vi "TEST_Garaje.vi"() -> ()   [LabVIEW 2019]
uses:
  <vilib>/MakerHub/LINX/Public/Peripherals/Digital/Digital Read N Chans.vi
  <vilib>/MakerHub/LINX/Public/Peripherals/Digital/Digital Write N Chans.vi
  <vilib>/MakerHub/LINX/Public/Peripherals/Analog/Analog Read 1 Chan.vi
  <vilib>/MakerHub/LINX/Private/Local IO/LinxDigitalRead.vi
  <vilib>/MakerHub/LINX/Public/Utilities/Check Channel.vi
  <vilib>/MakerHub/LINX/Private/Local IO/LinxDigitalWrite.vi
  <vilib>/MakerHub/LINX/Public/Peripherals/Analog/Analog Read N Chans.vi
  <vilib>/MakerHub/LINX/Private/Local IO/LinxAnalogRead.vi
  <vilib>/MakerHub/LINX/Public/Utilities/Open Serial.vi
  <vilib>/MakerHub/LINX/Public/Sensors/Motion/Servo/Servo Open One Channel.vi
  <vilib>/MakerHub/LINX/Private/Utilties/Generate Error.vi
  <vilib>/MakerHub/LINX/Public/Sensors/Motion/Servo/Servo Set Pulse Width One Channel.vi
  <vilib>/MakerHub/LINX/Public/Sensors/Motion/Servo/Servo Close One Channel.vi
  <vilib>/MakerHub/LINX/LMH-LINX.lvlib
  <vilib>/MakerHub/LINX/Public/Sensors/Motion/Servo/Servo.lvlib
panel:
  out "Slide 2":dbl(slide) scale=0.0..5.0
  out "Voltaje LDR":dbl
  out "ROJO":bool
  out "VERDE":bool
  in  "Serial Port":refnum<visa-resource-name>
  out "Loop Rate (Hz)":u32
  in  "Abrir":bool
  in  "Cerrar":bool
  in  "Stop Button":bool
  out "Slide":i32(slide) scale=0.0..100.0
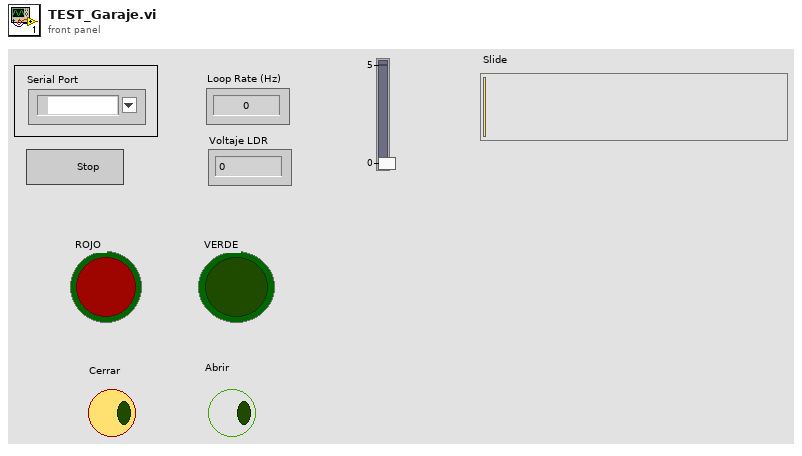
[diagram p1: front panel]
types:
  T1 = typedef "LMH-LINX.lvlib/LINX Ref.ctl" = cluster{"IO":T2, "Interface":T3, "LINX Device Config":T4}
  T2 = typedef "LMH-LINX.lvlib/Platform.ctl" = enum16{"Remote", "Local"}
  T3 = typedef "LMH-LINX.lvlib/Interface.ctl" = enum16{"Serial", "TCP"}
  T4 = typedef "LMH-LINX.lvlib/Device.lvlib/LINX Device Config.ctl" = cluster{"Interface":T3, "COM Port":refnum<visa-resource-name>, "TCP Configuration":T5, "Device Family":u8, "Device ID":u8, "Device Name":string, "TCP Ref":refnum<k5>, "Channels":T6}
  T5 = typedef "LMH-LINX.lvlib/Device.lvlib/TCP Config.ctl" = cluster{"IP Address":string, "Port":u16}
  T6 = typedef "LMH-LINX.lvlib/Channels.ctl" = cluster{"DI":u8[], "DO":u8[], "AI":u8[], "AO":u8[], "PWM":u8[], "QE":u8[], "UART":u8[], "I2C 2":u8[], "SPI":u8[], "CAN":u8[], "Servo":u8[], "AI Ref (V)":dbl, "AI Resolution (Bits)":u8, "AO Ref (V)":dbl, "AO Resolution (Bits)":u8}
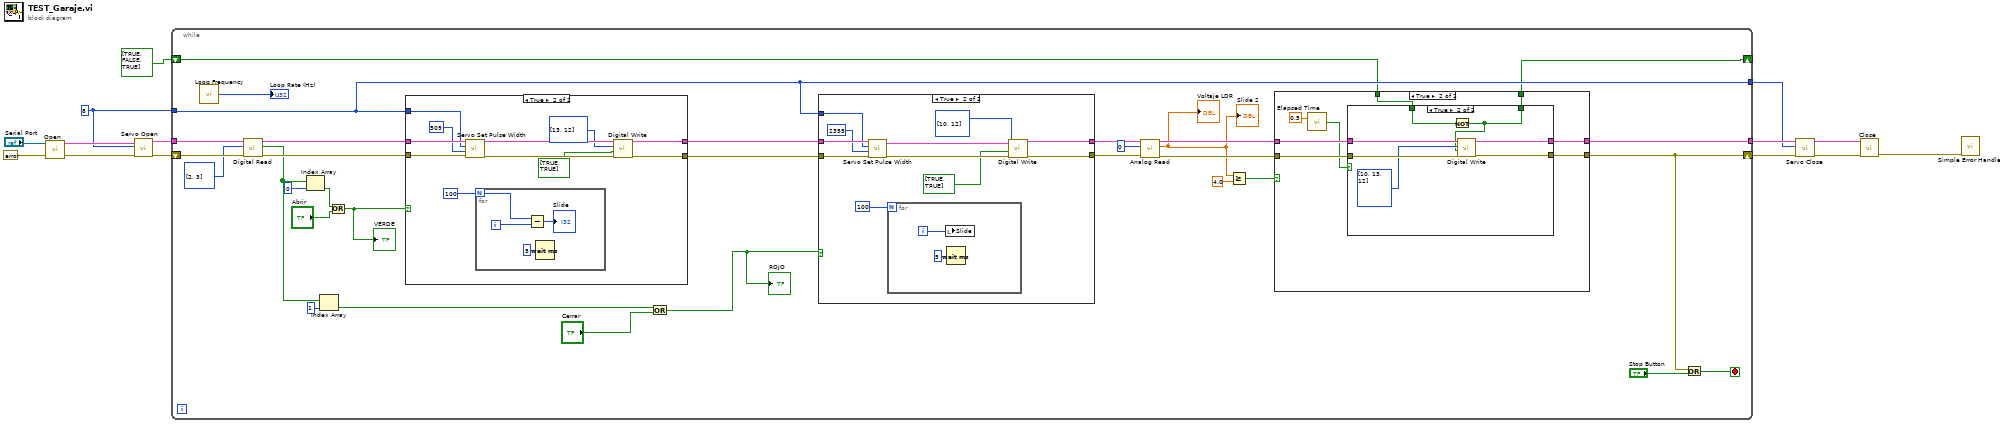
[diagram p0: block diagram]
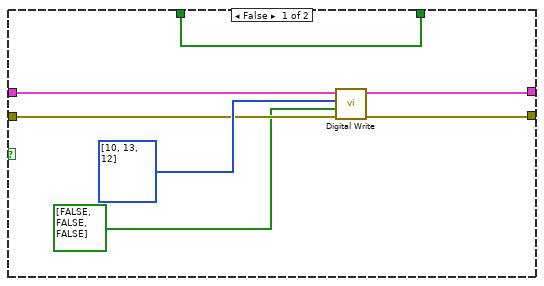
[diagram p2: hidden frame]
diagram:
  w4 = u8 8 ("Servo Channel")
  n1 = call-poly <vilib>:"Open.vi"("Error In"=errorcluster {"status"=FALSE, "code"=0, "source"=""}, "Serial Port"="Serial Port") -> ("Error Out"=w3:errorcluster, "LINX Resource"=w6:T1)  [unwired: 7 in, 1 out]
  n2 = call-poly <vilib>:"Servo Open.vi"("Error In"=w3, "Servo Channel"=w4, "LINX Resource"=w6) -> ("Error Out"=w2:errorcluster, "LINX Resource"=w5:T1)  [unwired: 7 in]
  n3 = while {
    tunnel: w5 -> [w39]
    shift-right: [w19] -> w10
    shift-left: w2 -> [w40]
    tunnel: w4 -> [w41]
    tunnel: [w20] -> w11
    tunnel: [w41] -> w7
    shift-right: [w16] -> _
    shift-left: bool[] [TRUE, FALSE, TRUE] ("Values") -> [w17]
    stop <- w46 stop-if-true
    n4 = call <vilib>:"Loop Frequency.vi"() -> ("Loop Rate (Hz)"=→"Loop Rate (Hz)":u32)
    n5 = call-poly <vilib>:"Digital Read.vi"("Error In"=w40, "DI Channels"=u8[] [2, 3] ("Array"), "LINX Resource"=w39) -> ("Error Out"=w37:errorcluster, "Values"=w32:bool[], "LINX Resource"=w38:T1)  [unwired: 6 in]
    n6 = Index Array "Index Array"(array=w32, index=0) -> (element=w33:bool)
    n7 = Index Array "Index Array"(array=w32, index=1) -> (element=w30:bool)
    n8 = Or(x=w33, y="Abrir") -> (x .or. y?=w28:bool)
    "VERDE" <- w28
    n9 = case shown="True" w28 {
      tunnel: w37 -> [w87 w99]
      tunnel: [w87 w92] -> w43
      tunnel: w38 -> [w88 w98]
      tunnel: [w88 w93] -> w42
      tunnel: w41 -> [_ w97]
      frame False {
      }
      frame True {
        n10 = call-poly <vilib>:"Servo Set Pulse Width.vi"("Error In"=w99, "Pulse Width (uS)"=509, "Servo Channel"=w97, "LINX Resource"=w98) -> ("Error Out"=w94:errorcluster, "LINX Resource"=w95:T1)  [unwired: 6 in]
        n11 = for {
          N: 100 -> [w103]
          i -> [w102]
          n12 = Subtract(x=w103, y=w102) -> (x-y=→"Slide":i32)
          n13 = Wait (ms)(milliseconds to wait=u32 5) -> ()  [unwired: 1 out]
        }
        n14 = call-poly <vilib>:"Digital Write.vi"("Error In"=w94, "Values"=bool[] [TRUE, TRUE], "DO Channels"=u8[] [13, 12], "LINX Resource"=w95) -> ("Error Out"=w92:errorcluster, "LINX Resource"=w93:T1)  [unwired: 6 in]
      }
    }
    n15 = Or(x=w30, y="Cerrar") -> (x .or. y?=w27:bool)
    "ROJO" <- w27
    n16 = case shown="True" w27 {
      tunnel: w43 -> [w72 w84]
      tunnel: [w72 w78] -> w25
      tunnel: w42 -> [w73 w83]
      tunnel: [w73 w77] -> w26
      tunnel: w41 -> [_ w82]
      frame False {
      }
      frame True {
        n17 = call-poly <vilib>:"Servo Set Pulse Width.vi"("Error In"=w84, "Pulse Width (uS)"=2355, "Servo Channel"=w82, "LINX Resource"=w83) -> ("Error Out"=w79:errorcluster, "LINX Resource"=w80:T1)  [unwired: 6 in]
        n18 = for {
          N: u8 100 ("Slide") -> [_]
          i -> [w85]
          n19 = local write "Slide"(w85) -> ()
          n20 = Wait (ms)(milliseconds to wait=u32 5) -> ()  [unwired: 1 out]
        }
        n21 = call-poly <vilib>:"Digital Write.vi"("Error In"=w79, "Values"=bool[] [TRUE, TRUE], "DO Channels"=u8[] [10, 12], "LINX Resource"=w80) -> ("Error Out"=w78:errorcluster, "LINX Resource"=w77:T1)  [unwired: 6 in]
      }
    }
    n22 = call-poly <vilib>:"Analog Read.vi"("Error In"=w25, "Analog Channel"=u8 0, "LINX Resource"=w26) -> ("Error Out"=w21:errorcluster, "Voltage"=w18:dbl, "LINX Resource"=w22:T1)  [unwired: 5 in, 1 out]
    "Voltaje LDR" <- w18
    "Slide 2" <- w18
    n23 = Greater Or Equal?(x=w18, y=4.0) -> (x >= y?=w15:bool)
    n24 = case shown="True" w15 {
      tunnel: w22 -> [w50 w60]
      tunnel: w21 -> [w51 w61]
      tunnel: [w49 w59] -> w20
      tunnel: [w48 w58] -> w19
      tunnel: w17 -> [w53 w57]
      tunnel: [w53 w56] -> w16
      frame False {
        n25 = call-poly <vilib>:"Digital Write.vi"("Error In"=w51, "Values"=bool[] [FALSE, FALSE, FALSE], "DO Channels"=u8[] [10, 13, 12] ("Array"), "LINX Resource"=w50) -> ("Error Out"=w48:errorcluster, "LINX Resource"=w49:T1)  [unwired: 6 in]
      }
      frame True {
        n26 = call "Elapsed Time"("Time Target (s)"=0.5) -> ("Time has Elapsed"=w54:bool)  [unwired: 11 in, 7 out]
        n27 = case shown="True" w54 {
          tunnel: w61 -> [w62 w71]
          tunnel: w60 -> [w63 w70]
          tunnel: [w63 w69] -> w59
          tunnel: [w62 w68] -> w58
          tunnel: w57 -> [w64 w66]
          tunnel: [w64 w65] -> w56
          frame False {
          }
          frame True {
            n28 = Not(x=w66) -> (.not. x?=w65:bool[])
            n29 = call-poly <vilib>:"Digital Write.vi"("Error In"=w71, "Values"=w65, "DO Channels"=u8[] [10, 13, 12] ("Array"), "LINX Resource"=w70) -> ("Error Out"=w68:errorcluster, "LINX Resource"=w69:T1)  [unwired: 6 in]
          }
        }
      }
    }
    n30 = Or(x=w19, y="Stop Button") -> (x .or. y?=w46:bool)
  }
  n31 = call-poly <vilib>:"Servo Close.vi"("Error In"=w10, "Servo Channel"=w7, "LINX Resource"=w11) -> ("Error Out"=w9:errorcluster, "LINX Resource"=w8:T1)  [unwired: 7 in]
  n32 = call <vilib>:"Close.vi"("Error In"=w9, "LINX Resource"=w8) -> ("Error Out"=w14:errorcluster)  [unwired: 9 in]
  n33 = call <vilib>:"Simple Error Handler.vi"("error in (no error)"=w14) -> ()  [unwired: 4 in, 5 out]
